vi "Cleanup.vi"(8 "error in (no error)":errorcluster, 11 "Message Scripter in":refnum<class "Message Scripter.lvclass">) -> (0 "error out":errorcluster, 3 "Message Scripter out":refnum<class "Message Scripter.lvclass">)   [LabVIEW 2020, in "Message Maker.lvlib" / "Message Scripter.lvclass"]
uses:
  Message Scripter.lvclass
  Prototyper/Prototyper.lvclass
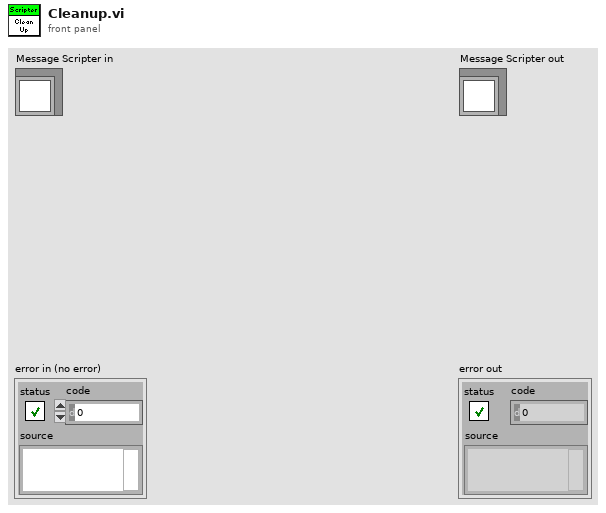
[diagram p1: front panel]
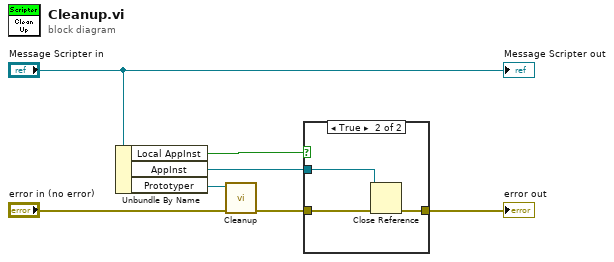
[diagram p0: block diagram]
diagram:
  n1 = Unbundle By Name("Message Scripter in") -> ("Local AppInst"=w1:bool, "AppInst"=w2:refnum<vi>, "Prototyper"=w4:refnum<class "Prototyper.lvclass">)
  n2 = call-dynamic "Cleanup.vi"("error in (no error)"="error in (no error)", "Prototyper in"=w4) -> ("error out"=w6:errorcluster)  [unwired: 8 in, 1 out]
  n3 = case shown="True" w1 {
    tunnel: w6 -> [w8 w11]
    tunnel: [w8 w10] -> w3
    tunnel: w2 -> [_ w9]
    frame False {
    }
    frame True {
      n4 = Close Reference(reference=w9, error in (no error)=w11) -> (error out=w10:errorcluster)
    }
  }
  "error out" <- w3
  "Message Scripter out" <- "Message Scripter in"
